vi "add units.vi"(7 "Language":string, 9 "Array":dbl[](array[numeric]), 10 "Numeric":dbl, 11 "Label Text":string) -> (1 "Converted Array":dbl[](array[numeric]), 2 "Converted Numeric":dbl, 3 "unit in brackets":string, 4 "format string":string, 5 "unit":string)   [LabVIEW 2012, in "Design Server.lvlib"]
uses:
  Design Server.lvlib
panel:
  # "Et\tEntrance Tank\tformerly grit chamber\nAmp\tamplitude\tL\nB\tperpendicular distance between components (center to center)\tL\nE\tpipe roughness\tL\nFB\tFreeboard\tL\nH\theight (includes freeboard)\tL\nHL\thead loss\tL\nHW\tlocal water depth\tL\nID\tinner diameter\tL\nL\tlength\tL\nLoc\tLocations\tL\nND\tnominal diameter\tL\nOD\touter diameter\tL\nR\tRadius\tL\nS\tspace between components\tL\nT\tthickness\tL\nW\twidth\tL\nZ\televation relative to bottom of sed tank\tL\nZW\twater depth relative to bottom of sed tank\tL\nV\tvelocity\tL/T\nCP\tCollision Potential\tL^(2/3)\nA\tArea\tL^2\nNu\tkinematic viscosity\tL^2/T\nED\tenergy dissipation rate\tL^2/T^3\nVol\tvolume\tL^3\nQ\tflow\tL^3/T\nMW\tMolecular weight\tM\nC\tConcentration\tM/L^3\nRho\tDensity\tM/L^3\nAN\tangle\tradians\nTi\ttime\tT"
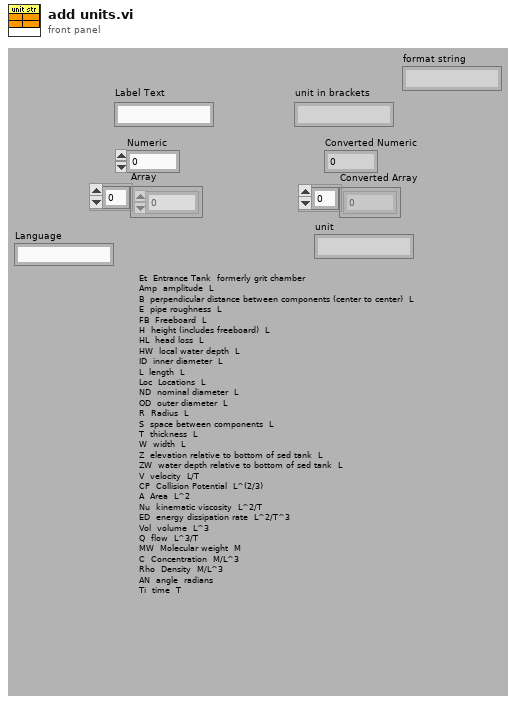
[diagram p1: front panel]
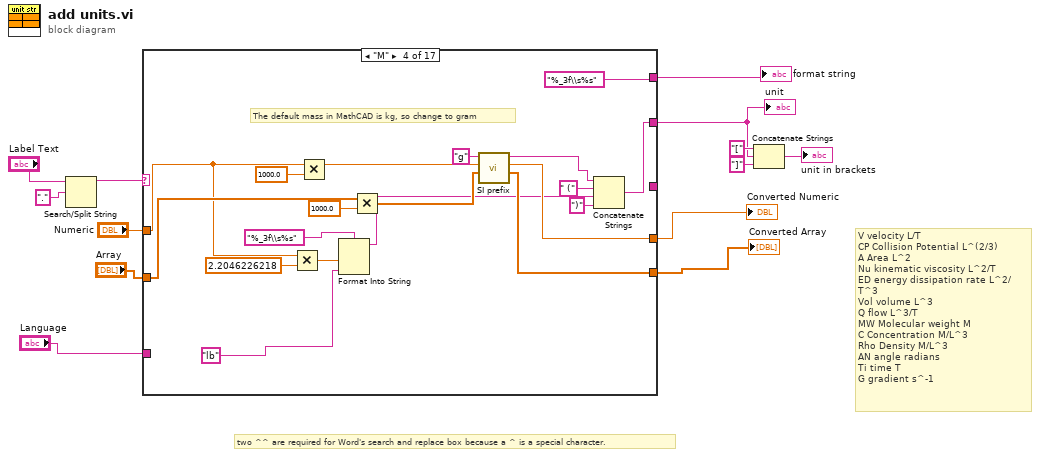
[diagram p0: block diagram]
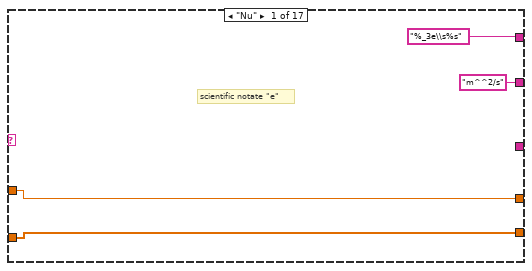
[diagram p2: hidden frame]
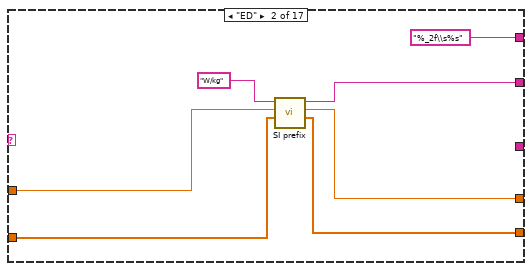
[diagram p3: hidden frame]
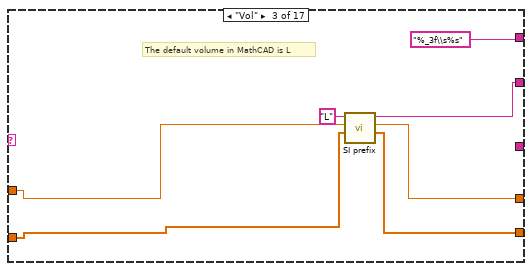
[diagram p4: hidden frame]
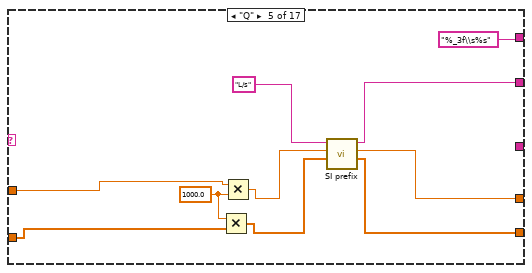
[diagram p5: hidden frame]
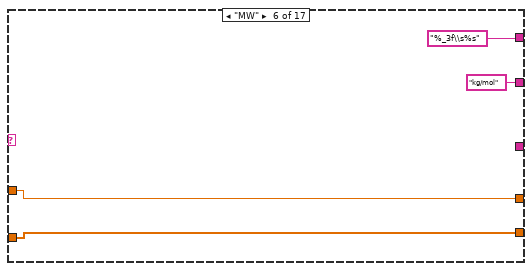
[diagram p6: hidden frame]
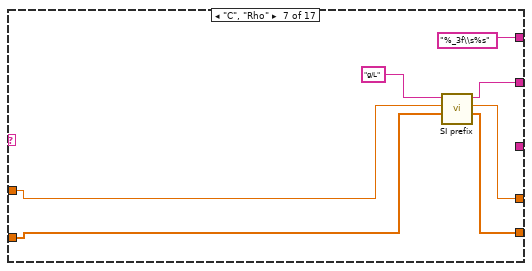
[diagram p7: hidden frame]
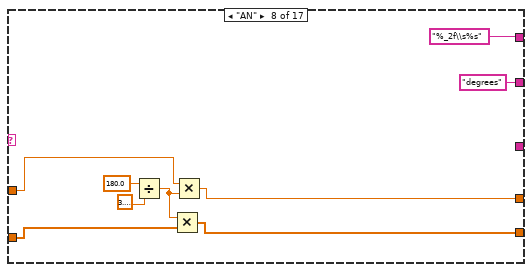
[diagram p8: hidden frame]
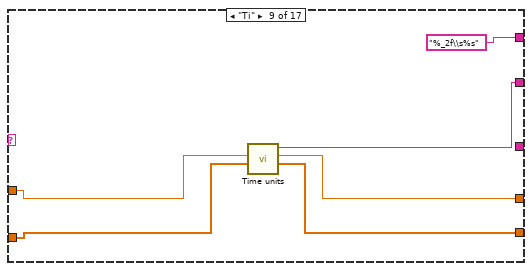
[diagram p9: hidden frame]
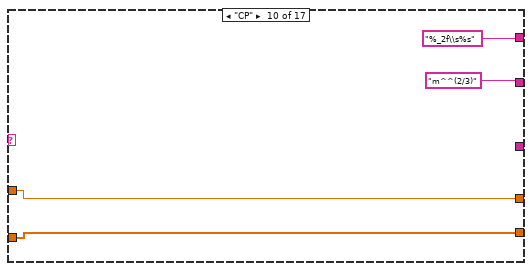
[diagram p10: hidden frame]
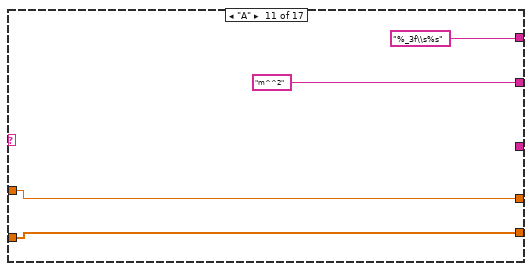
[diagram p11: hidden frame]
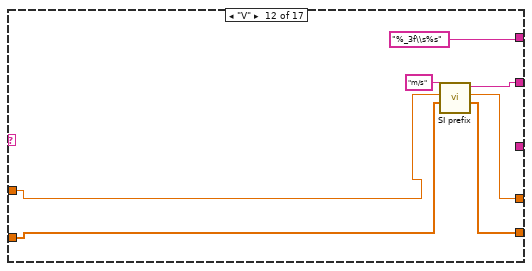
[diagram p12: hidden frame]
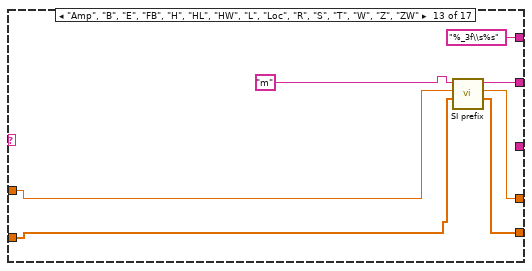
[diagram p13: hidden frame]
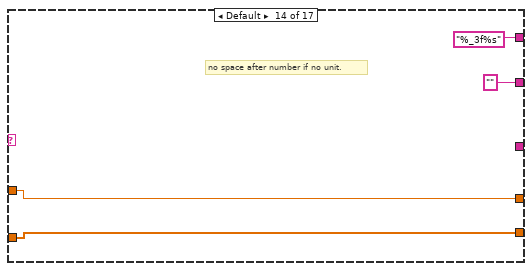
[diagram p14: hidden frame]
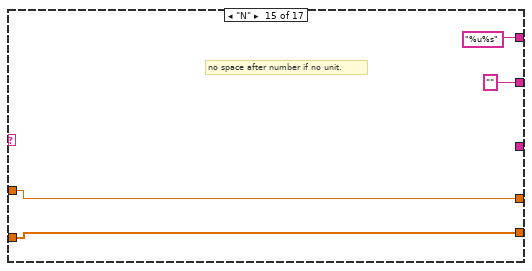
[diagram p15: hidden frame]
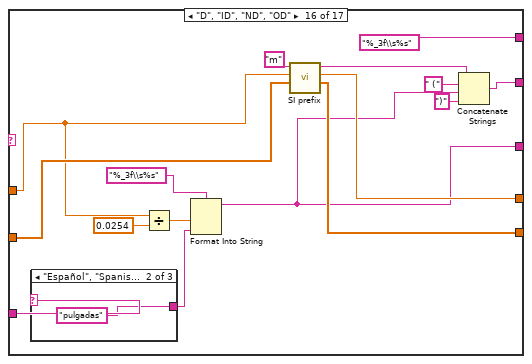
[diagram p16: hidden frame]
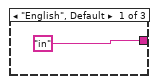
[diagram p17: hidden frame]
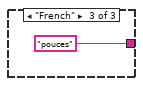
[diagram p18: hidden frame]
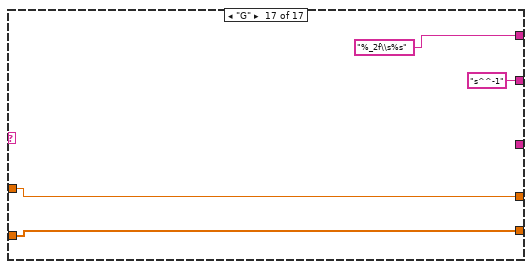
[diagram p19: hidden frame]
diagram:
  # "two ^^ are required for Word's search and replace box because a ^ is a special character."
  # "V\tvelocity\tL/T\nCP\tCollision Potential\tL^(2/3)\nA\tArea\tL^2\nNu\tkinematic viscosity\tL^2/T\nED\tenergy dissipation rate\tL^2/T^3\nVol\tvolume\tL^3\nQ\tflow\tL^3/T\nMW\tMolecular weight\tM\nC\tConcentration\tM/L^3\nRho\tDensity\tM/L^3\nAN\tangle\tradians\nTi\ttime\tT\nG gradient s^-1"
  n1 = Search/Split String(string="Label Text", search string/char (-)="." ("regular expression")) -> (substring before match=w11:string)  [unwired: 1 in, 2 out]
  n2 = case shown="\"M\"" w11 {
    tunnel: ["m^^2/s" w22 w25 w32 w55 "kg/mol" w69 "degrees" w81 "m^^(2/3)" "m^^2" w99 w106 "" "" w122 "s^^-1" ("modified unit")] -> w4
    tunnel: "Numeric" -> [w16 w21 w30 w37 w59 w63 w68 w76 w85 w89 w93 w96 w105 w111 w115 w128 w138]
    tunnel: "Array" -> [w15 w20 w29 w43 w58 w62 w66 w75 w84 w88 w92 w98 w103 w110 w114 w131 w137]
    tunnel: [w15 w18 w27 w48 w51 w62 w65 w73 w83 w88 w92 w97 w102 w110 w114 w130 w137] -> w2
    tunnel: [w16 w19 w28 w49 w53 w63 w67 w74 w82 w89 w93 w95 w104 w111 w115 w129 w138] -> w3
    tunnel: ["%_3e\\s%s" "%_2f\\s%s" "%_3f\\s%s" "%_3f\\s%s" "%_3f\\s%s" "%_3f\\s%s" "%_3f\\s%s" "%_2f\\s%s" "%_2f\\s%s" "%_2f\\s%s" "%_3f\\s%s" "%_3f\\s%s" "%_3f\\s%s" "%_3f%s" "%u%s" "%_3f\\s%s" "%_2f\\s%s"] -> w5
    tunnel: [_ _ _ _ _ _ _ _ _ _ _ _ _ _ _ w121 _] -> _
    tunnel: "Language" -> [_ _ _ _ _ _ _ _ _ _ _ _ _ _ _ w118 _]
    frame "Nu" {
      # "scientific notate \"e\""
    }
    frame "ED" {
      n3 = call "SI prefix.vi"("Array"=w20, "Numeric"=w21, "Unit"="W/kg") -> ("Scaled Array"=w18:dbl[], "Scaled Number"=w19:dbl, "modified unit"=w22:string)  [unwired: 6 in]
    }
    frame "Vol" {
      # "The default volume in MathCAD is L"
      n4 = call "SI prefix.vi"("Array"=w29, "Numeric"=w30, "Unit"="L") -> ("Scaled Array"=w27:dbl[], "Scaled Number"=w28:dbl, "modified unit"=w25:string)  [unwired: 6 in]
    }
    frame "M" {
      # "The default mass in MathCAD is kg, so change to gram"
      n5 = Multiply(x=w37, y=2.2046226218) -> (x*y=w40:dbl)
      n6 = Multiply(x=w37, y=1000.0) -> (x*y=w46:dbl)
      n7 = Format Into String(format string="%_3f\\s%s", w40, "lb") -> (resulting string=w34:string)  [unwired: 2 in, 1 out]
      n8 = Multiply(x=w43, y=1000.0) -> (x*y=w42:dbl[])
      n9 = call "SI prefix.vi"("Array"=w42, "Numeric"=w46, "Unit"="g") -> ("Scaled Array"=w48:dbl[], "Scaled Number"=w49:dbl, "modified unit"=w33:string)  [unwired: 6 in]
      n10 = Concatenate Strings(w33, " (" ("string"), w34, ")" ("string")) -> (w32:string)
    }
    frame "Q" {
      w60 = 1000.0 ("y")
      n11 = Multiply(x=w60, y=w58) -> (x*y=w52:dbl[])
      n12 = Multiply(x=w59, y=w60) -> (x*y=w54:dbl)
      n13 = call "SI prefix.vi"("Array"=w52, "Numeric"=w54, "Unit"="L/s") -> ("Scaled Array"=w51:dbl[], "Scaled Number"=w53:dbl, "modified unit"=w55:string)  [unwired: 6 in]
    }
    frame "MW" {
    }
    frame "C", "Rho" {
      n14 = call "SI prefix.vi"("Array"=w66, "Numeric"=w68, "Unit"="g/L") -> ("Scaled Array"=w65:dbl[], "Scaled Number"=w67:dbl, "modified unit"=w69:string)  [unwired: 6 in]
    }
    frame "AN" {
      n15 = Divide(x=180.0 ("y"), y=3.141592653589793) -> (x/y=w79:dbl)
      n16 = Multiply(x=w79, y=w75) -> (x*y=w73:dbl[])
      n17 = Multiply(x=w76, y=w79) -> (x*y=w74:dbl)
    }
    frame "Ti" {
      n18 = call "Time units.vi"("Array"=w84, "Numeric"=w85) -> ("Scaled Array"=w83:dbl[], "Scaled Number"=w82:dbl, "modified unit"=w81:string)  [unwired: 7 in]
    }
    frame "CP" {
    }
    frame "A" {
    }
    frame "V" {
      n19 = call "SI prefix.vi"("Array"=w98, "Numeric"=w96, "Unit"="m/s") -> ("Scaled Array"=w97:dbl[], "Scaled Number"=w95:dbl, "modified unit"=w99:string)  [unwired: 6 in]
    }
    frame "Amp", "B", "E", "FB", "H", "HL", "HW", "L", "Loc", "R", "S", "T", "W", "Z", "ZW" {
      n20 = call "SI prefix.vi"("Array"=w103, "Numeric"=w105, "Unit"="m") -> ("Scaled Array"=w102:dbl[], "Scaled Number"=w104:dbl, "modified unit"=w106:string)  [unwired: 6 in]
    }
    frame Default {
      # "no space after number if no unit."
    }
    frame "N" {
      # "no space after number if no unit."
    }
    frame "D", "ID", "ND", "OD" {
      n21 = case shown="\"Español\", \"Spanish\", \"español\", \"spanish\"" w118 {
        tunnel: ["in" ("input 2") "pulgadas" "pouces"] -> w117
        frame "English", Default {
        }
        frame "Español", "Spanish", "español", "spanish" {
        }
        frame "French" {
        }
      }
      n22 = Divide(x=w128, y=0.0254) -> (x/y=w126:dbl)
      n23 = Format Into String(format string="%_3f\\s%s", w126, w117) -> (resulting string=w121:string)  [unwired: 2 in, 1 out]
      n24 = call "SI prefix.vi"("Array"=w131, "Numeric"=w128, "Unit"="m") -> ("Scaled Array"=w130:dbl[], "Scaled Number"=w129:dbl, "modified unit"=w123:string)  [unwired: 6 in]
      n25 = Concatenate Strings(w123, " (" ("string"), w121, ")" ("string")) -> (w122:string)
    }
    frame "G" {
    }
  }
  "Converted Numeric" <- w3
  "Converted Array" <- w2
  "unit" <- w4
  "format string" <- w5
  n26 = Concatenate Strings("[" ("string"), w4, "]" ("string")) -> (→"unit in brackets":string)
